vi "Status Write Write Enable.vi"(8 "error in (no error)":errorcluster, 9 "WrEn":bool, 11 "Status Reference":T1) -> (0 "error out":errorcluster, 3 "Status Reference out":T1)   [LabVIEW 2021, in "Status.lvlib"]
uses:
  Status.lvlib
  Ctl/control.ctl
  Ctl/State.ctl
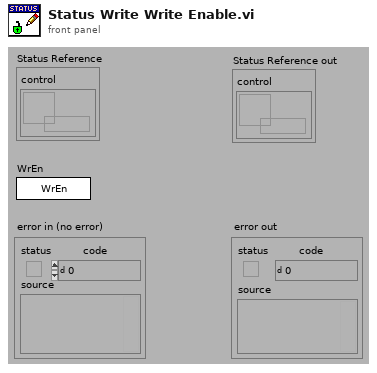
[diagram p1: front panel]
types:
  T1 = typedef "Status.lvlib/control.ctl" = cluster{"control":refnum<data-value>}
  T2 = typedef "Status.lvlib/State.ctl" = enum8{"initialization", "redefine", "standby", "connect", "wait to reconnect", "wait to reset timeout", "configure", "requests", "close connection", "stop"}
  T3 = cluster{"set_state":cluster{"Start":bool, "WrEn":bool, "Stop":bool}, "state":cluster{"errors":i32, "connect":bool, "state":T2}}
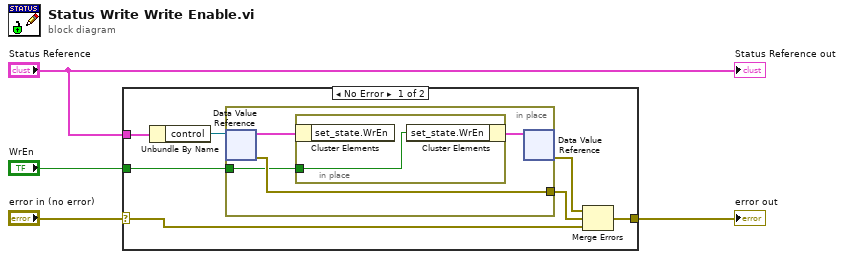
[diagram p0: block diagram]
diagram:
  n1 = case shown="No Error" "error in (no error)" {
    selector: "error in (no error)" -> [w5 w17]
    tunnel: [w10 w17] -> w1
    tunnel: "Status Reference" -> [w11 _]
    tunnel: "WrEn" -> [w9 _]
    frame No Error {
      n2 = Unbundle By Name(w11) -> ("control"=w6:refnum<data-value>)
      n3 = in-place {
        in-place-border: [w15] -> w7
        in-place-border: w9 -> [w13]
        n4 = in-place-dvr #1(w6) -> (w14:T3, w15:errorcluster)
        n5 = in-place {
          in-place-border: w13 -> [w16]
          n6 = in-place-cluster #2(w14) -> ()  [unwired: 1 out]
          n7 = in-place-cluster #2("set_state.WrEn"=w16) -> (w12:T3)
        }
        n8 = in-place-dvr #1(w12) -> (w8:errorcluster)  [unwired: 1 out]
      }
      n9 = Merge Errors(w8, w7, w5) -> (w10:errorcluster)
    }
    frame Error {
    }
  }
  "error out" <- w1
  "Status Reference out" <- "Status Reference"
